vi "Tab Example Code LV 2012.vi"() -> ()   [LabVIEW 2015]
panel:
  in  "Tab Control":enum32{"Page 1", "Page 2", "Page 3", "Page 4"}(tab)
  in  "stop 2":bool
  out "Numeric":dbl
  out "Boolean":bool
  in  "Toggle":bool
  in  "Button 1":bool
  in  "Button 4":bool
  in  "Button 3":bool
  in  "Button 2":bool
  in  "stop":bool
  # "Count until new tab is selected"
  # "On"
  # "Off"
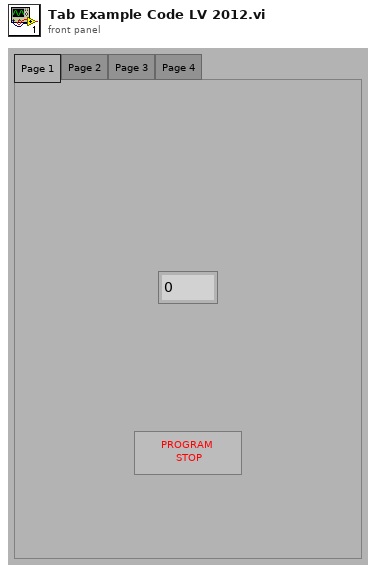
[diagram p1: front panel]
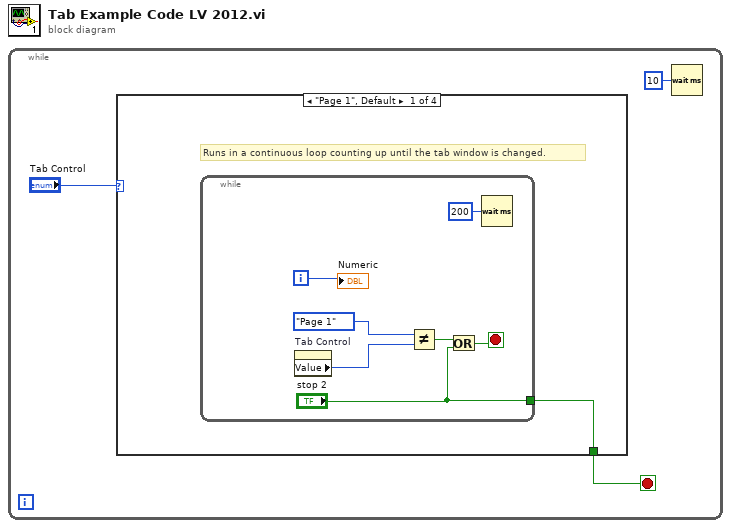
[diagram p0: block diagram]
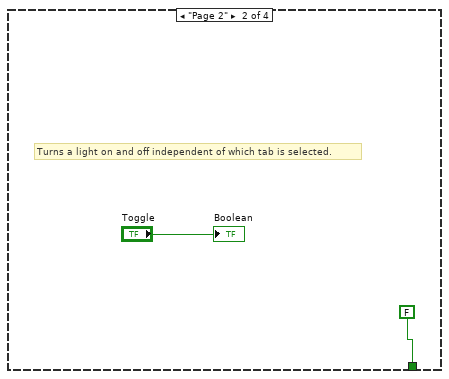
[diagram p2: hidden frame]
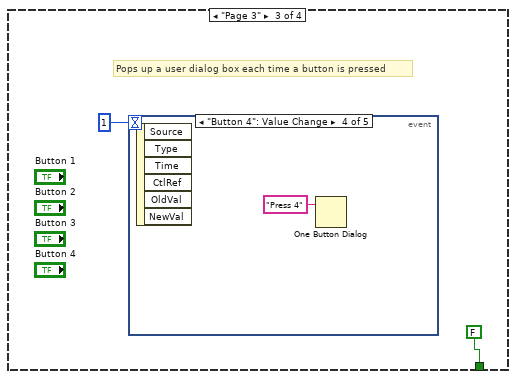
[diagram p3: hidden frame]
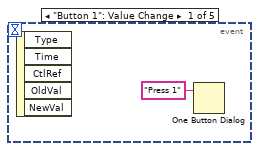
[diagram p4: hidden frame]
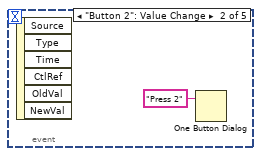
[diagram p5: hidden frame]
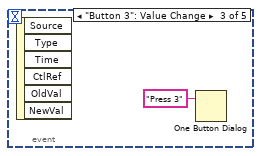
[diagram p6: hidden frame]
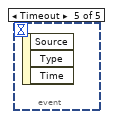
[diagram p7: hidden frame]
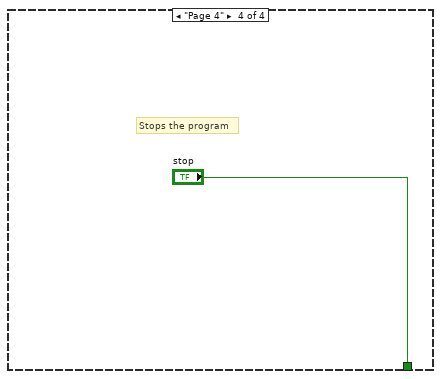
[diagram p8: hidden frame]
diagram:
  n1 = while {
    stop <- w2 stop-if-true
    n2 = case shown="\"Page 1\", Default" "Tab Control" {
      tunnel: [w4 FALSE ("stop") FALSE ("stop") "stop"] -> w2
      frame "Page 1", Default {
        # "Runs in a continuous loop counting up until the tab window is changed."
        n3 = while {
          tunnel: ["stop 2"] -> w4
          i -> [w11]
          stop <- w6 stop-if-true
          n4 = property on="Tab Control" class="TabCtl (strict)"() -> ("Value"=w7:enum32{"Page 1", "Page 2", "Page 3", "Page 4"})  [unwired: 2 in, 2 out]
          n5 = Not Equal?(x=enum32{"Page 1", "Page 2", "Page 3", "Page 4"}."Page 1" ("Tab Control 2"), y=w7) -> (x != y?=w8:bool)
          n6 = Or(x=w8, y="stop 2") -> (x .or. y?=w6:bool)
          n7 = Wait (ms)(milliseconds to wait=u32 200) -> ()  [unwired: 1 out]
          "Numeric" <- w11
        }
      }
      frame "Page 2" {
        # "Turns a light on and off independent of which tab is selected."
        "Boolean" <- "Toggle"
      }
      frame "Page 3" {
        # "Pops up a user dialog box each time a button is pressed"
        n8 = event shown="[3] \"Button 4\": Value Change" {
          selector: _ -> [_ _ _ _ _]
          dyn-events: _ -> [_ _ _ _ _]
          timeout: 1 -> [_ _ _ _ _]
          event "Button 1": Value Change {
            n9 = event-data() -> ()  [unwired: 6 out]
            n10 = One Button Dialog(message="Press 1") -> ()  [unwired: 2 out]
          }
          event "Button 2": Value Change {
            n11 = event-data() -> ()  [unwired: 7 out]
            n12 = One Button Dialog(message="Press 2") -> ()  [unwired: 2 out]
          }
          event "Button 3": Value Change {
            n13 = event-data() -> ()  [unwired: 7 out]
            n14 = One Button Dialog(message="Press 3") -> ()  [unwired: 2 out]
          }
          event "Button 4": Value Change {
            n15 = event-data() -> ()  [unwired: 7 out]
            n16 = One Button Dialog(message="Press 4") -> ()  [unwired: 2 out]
          }
          event Timeout {
            n17 = event-data() -> ()  [unwired: 4 out]
          }
        }
      }
      frame "Page 4" {
        # "Stops the program"
      }
    }
    n18 = Wait (ms)(milliseconds to wait=u32 10) -> ()  [unwired: 1 out]
  }
